vi "BK Precision 911X Series Run List Program.vi"() -> ()   [LabVIEW 2020]
doc: "This example demonstrates how to run a list program."
uses:
  BK Precision 911X Series.lvlib
panel:
  out "Actual Power Level (W)":dbl format="%.4g"
  out "Actual Voltage Level (V)":dbl format="%.4g"
  out "Actual Current Level (A)":dbl format="%.4g"
  in  "Stop List Program":bool
  in  "List Number (1)":dbl=1.0 min=1.0 max=10.0 format="%#_0f"
  in  "VISA resource name":refnum<visa-resource-name>
  # "(c) 2013 B&K Precision Corporation.  ALL RIGHTS RESERVED."
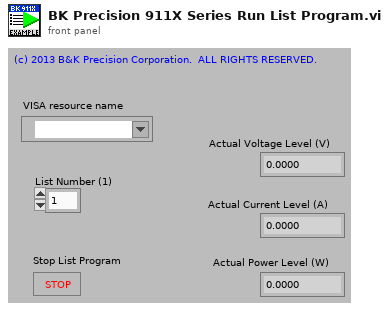
[diagram p1: front panel]
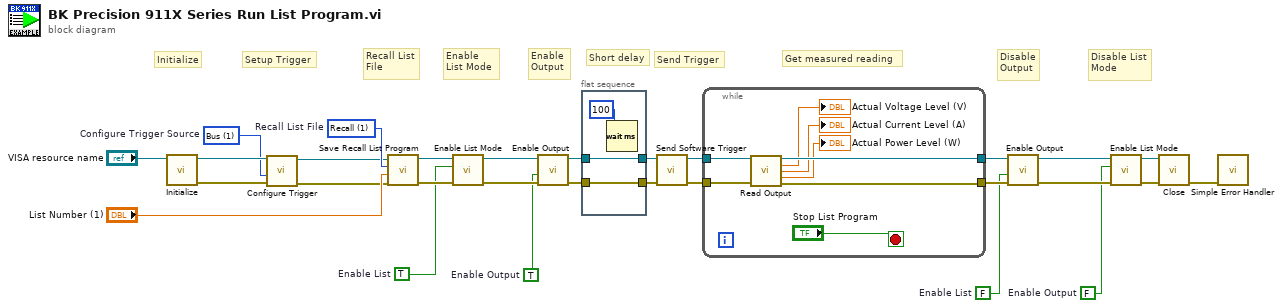
[diagram p0: block diagram]
diagram:
  w5 = u16 1 items=["Manual", "Bus"]  # Configure Trigger Source
  w10 = FALSE  # Enable Output
  w11 = FALSE  # Enable List
  w12 = TRUE  # Enable Output
  w13 = TRUE  # Enable List
  w27 = u16 1 items=["Save", "Recall"]  # Recall List File
  # "Short delay"
  # "Setup Trigger"
  # "Initialize"
  # "Disable List\nMode"
  # "Disable\nOutput"
  # "Recall List\nFile"
  # "Enable\nList Mode"
  # "Enable\nOutput"
  # "Send Trigger"
  # "Get measured reading"
  n1 = call "Initialize.vi"("VISA resource name"="VISA resource name") -> ("error out"=w6:errorcluster, "VISA resource name out"=w9:refnum<visa-resource-name>)  [unwired: 9 in]
  n2 = call "Configure Trigger.vi"("error in (no error)"=w6, "Trigger Source (0:Manual)"=w5, "VISA resource name"=w9) -> ("error out"=w7:errorcluster, "VISA resource name out"=w8:refnum<visa-resource-name>)  [unwired: 7 in]
  n3 = call "Save Recall List Program.vi"("error in (no error)"=w7, "List Number (1)"="List Number (1)", "Save Recall List File (0:Save)"=w27, "VISA resource name"=w8) -> ("error out"=w24:errorcluster, "VISA resource name out"=w25:refnum<visa-resource-name>)  [unwired: 6 in]
  n4 = call "Enable List Mode.vi"("error in (no error)"=w24, "Enable List Mode (F: False)"=w13, "VISA resource name"=w25) -> ("error out"=w22:errorcluster, "VISA resource name out"=w23:refnum<visa-resource-name>)  [unwired: 7 in]
  n5 = call "Enable Output.vi"("error in (no error)"=w22, "Enable Output (F: False)"=w12, "VISA resource name"=w23) -> ("error out"=w2:errorcluster, "VISA resource name out"=w3:refnum<visa-resource-name>)  [unwired: 7 in]
  n6 = flat-sequence {
    tunnel: [w32] -> w4
    tunnel: w3 -> [w32]
    tunnel: w2 -> [w31]
    tunnel: [w31] -> w1
    frame #0 {
      n7 = Wait (ms)(milliseconds to wait=100) -> ()  [unwired: 1 out]
    }
  }
  n8 = call "Send Software Trigger.vi"("error in (no error)"=w1, "VISA resource name"=w4) -> ("error out"=w14:errorcluster, "VISA resource name out"=w17:refnum<visa-resource-name>)  [unwired: 8 in]
  n9 = while {
    tunnel: w17 -> [w39]
    tunnel: [w36] -> w16
    tunnel: [w37] -> w15
    tunnel: w14 -> [w38]
    stop <- "Stop List Program" stop-if-true
    n10 = call "Read Output.vi"("VISA resource name"=w39, "error in (no error)"=w38) -> ("VISA resource name out"=w36:refnum<visa-resource-name>, "Actual Voltage Level (V)"=→"Actual Voltage Level (V)":dbl, "Actual Current Level (A)"=→"Actual Current Level (A)":dbl, "Actual Power Level (W)"=→"Actual Power Level (W)":dbl, "error out"=w37:errorcluster)  [unwired: 8 in, 1 out]
  }
  n11 = call "Enable Output.vi"("error in (no error)"=w15, "Enable Output (F: False)"=w11, "VISA resource name"=w16) -> ("error out"=w18:errorcluster, "VISA resource name out"=w19:refnum<visa-resource-name>)  [unwired: 7 in]
  n12 = call "Enable List Mode.vi"("error in (no error)"=w18, "Enable List Mode (F: False)"=w10, "VISA resource name"=w19) -> ("error out"=w21:errorcluster, "VISA resource name out"=w20:refnum<visa-resource-name>)  [unwired: 7 in]
  n13 = call "Close.vi"("error in (no error)"=w21, "VISA resource name"=w20) -> ("error out"=w28:errorcluster)  [unwired: 9 in]
  n14 = call <vilib>:"Simple Error Handler.vi"("error in (no error)"=w28) -> ()  [unwired: 4 in, 5 out]
